vi "Rio_Motor_Setpoint_Ramp.vi"(8 "Loop Count (t)":i64, 9 "Current Position":i64, 11 "Setpoint":dbl) -> (3 "Setpoint Sigmoid Function":dbl)   [LabVIEW 2017]
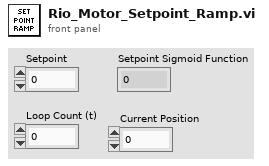
[diagram p1: front panel]
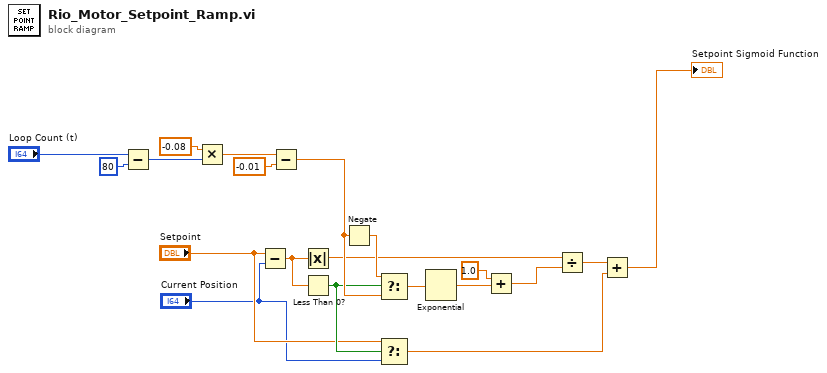
[diagram p0: block diagram]
diagram:
  n1 = Subtract(x="Loop Count (t)", y=80) -> (x-y=w16:i64)
  n2 = Multiply(x=-0.08, y=w16) -> (x*y=w19:dbl)
  n3 = Subtract(x="Setpoint", y="Current Position") -> (x-y=w11:dbl)
  n4 = Subtract(x=w19, y=-0.01) -> (x-y=w9:dbl)
  n5 = Absolute Value(x=w11) -> (abs(x)=w7:dbl)
  n6 = Less Than 0?(x=w11) -> (x < 0?=w4:bool)
  n7 = Negate(x=w9) -> (-x=w10:dbl)
  n8 = Select(t=w10, s=w4, f=w9) -> (s? t:f=w8:dbl)
  n9 = Select(t="Setpoint", s=w4, f="Current Position") -> (s? t:f=w2:dbl)
  n10 = Exponential(1:w8) -> (0:w14:dbl)
  n11 = Add(x=1.0, y=w14) -> (x+y=w13:dbl)
  n12 = Divide(x=w7, y=w13) -> (x/y=w6:dbl)
  n13 = Add(x=w6, y=w2) -> (x+y=→"Setpoint Sigmoid Function":dbl)
